vi "EditBluetoothValues.vi"(11 "In array":T1(array[cluster])) -> (3 "Out array":T1(array[cluster]))   [LabVIEW 2013, in "main.lvlib"]
uses:
  main.lvlib
panel:
  in  "EditBluetoothValuesBtn":bool
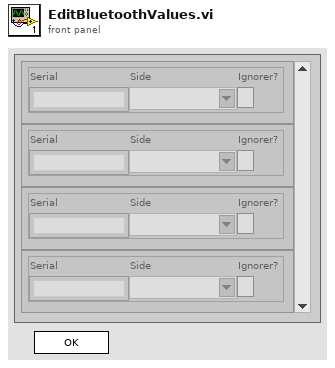
[diagram p1: front panel]
types:
  T1 = cluster{"Serial":string, "Side":string, "Ignorer?":bool}[]
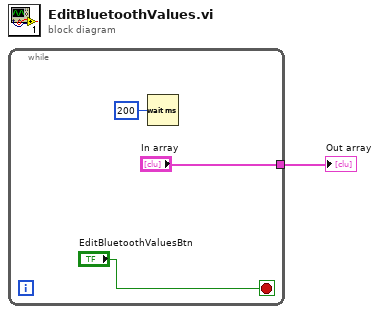
[diagram p0: block diagram]
diagram:
  n1 = while {
    tunnel: ["In array"] -> w1
    stop <- "EditBluetoothValuesBtn" stop-if-true
    n2 = Wait (ms)(milliseconds to wait=u32 200) -> ()  [unwired: 1 out]
  }
  "Out array" <- w1
